vi "23384_Davis_Poku_Amankwa_Amankwa.DavisPoku.MNE1201.7.1_348263_723397803.vi"() -> ()   [LabVIEW 2018]
panel:
  out "C":bool
  out "B":bool
  out "E":bool
  out "D":bool
  out "G":bool
  out "F":bool
  out "A":bool
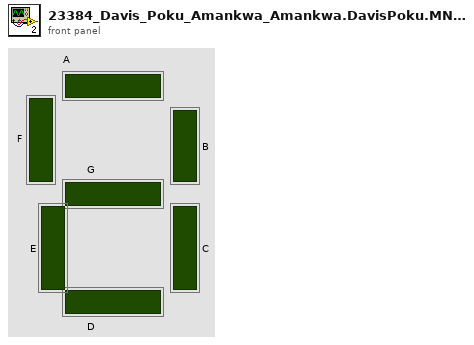
[diagram p1: front panel]
types:
  T1 = enum16{"0", "1", "2", "3", "4", "5", "6", "7", "8", "9", "OFF"}
  T2 = enum16{"0", "1", "2", "3", "4", "5", "6", "7", "8", "9"}
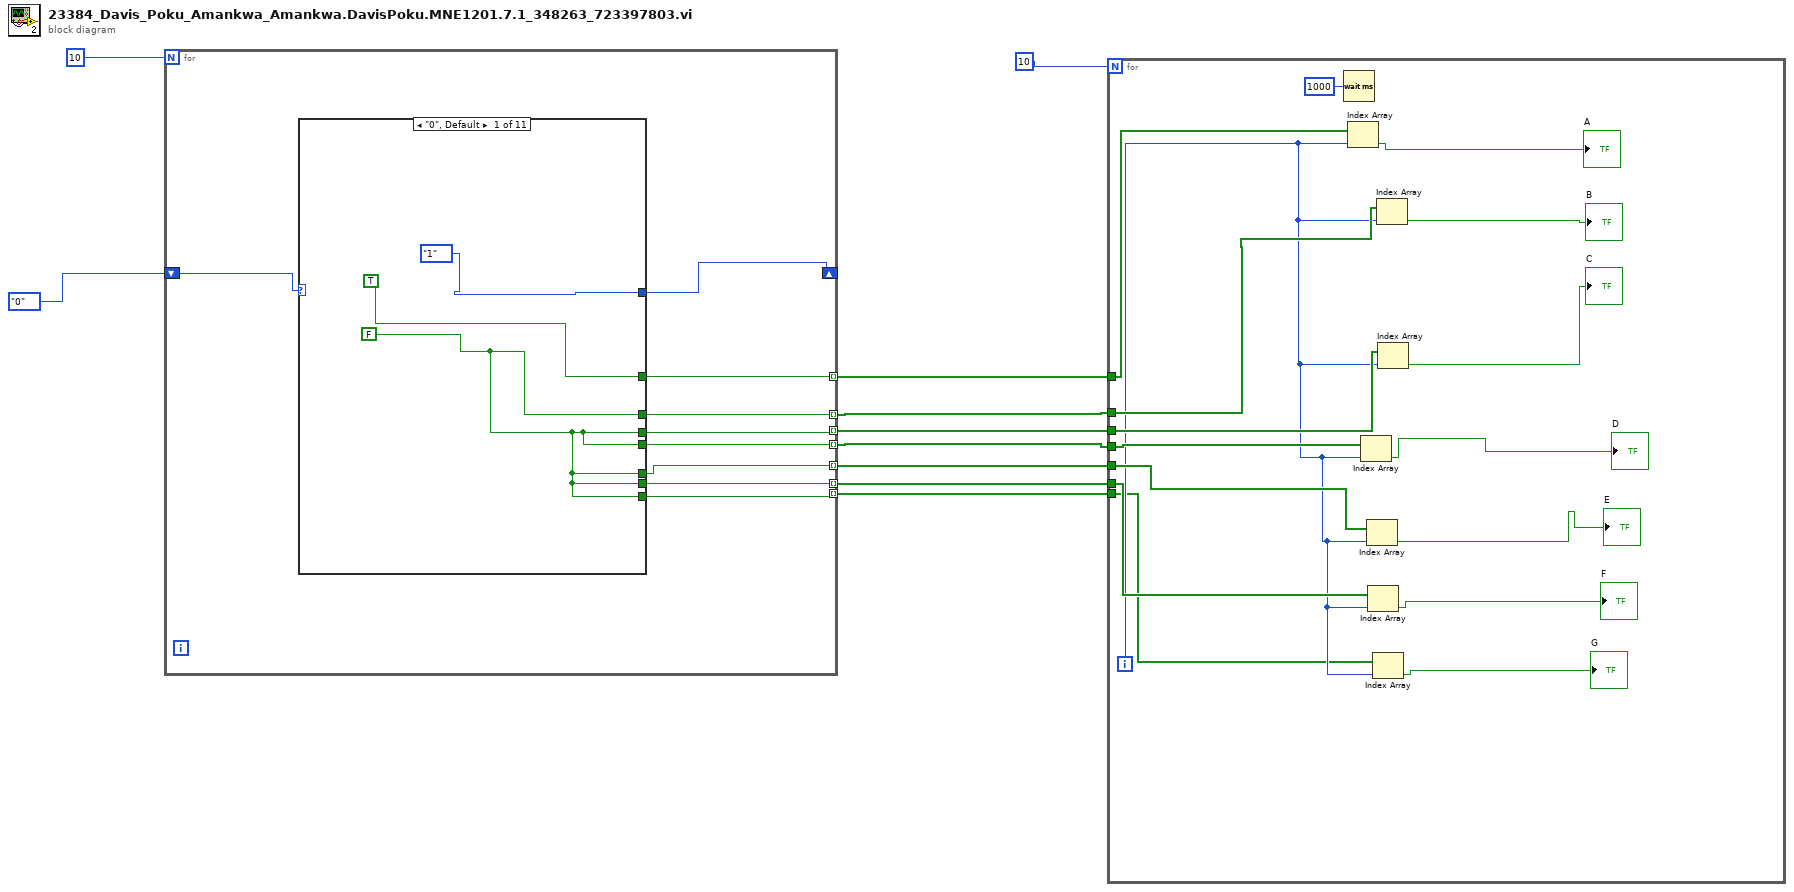
[diagram p0: block diagram]
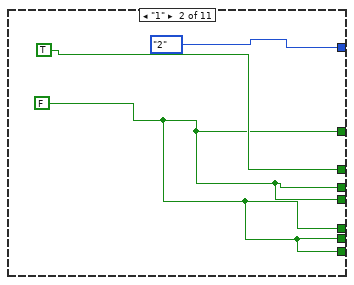
[diagram p2: hidden frame]
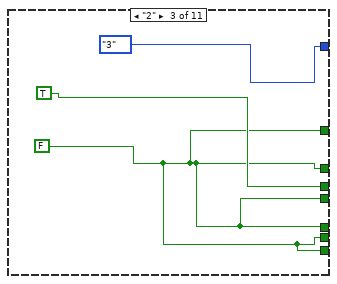
[diagram p3: hidden frame]
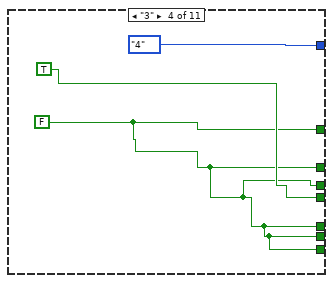
[diagram p4: hidden frame]
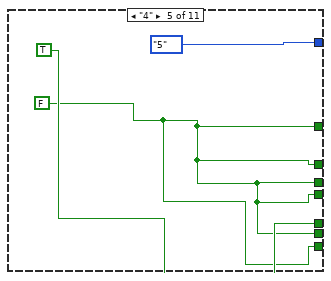
[diagram p5: hidden frame]
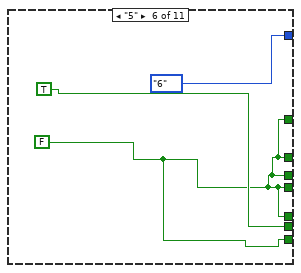
[diagram p6: hidden frame]
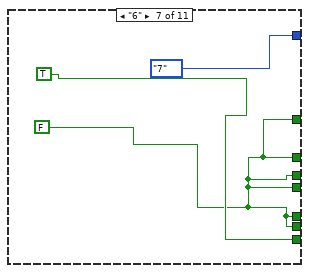
[diagram p7: hidden frame]
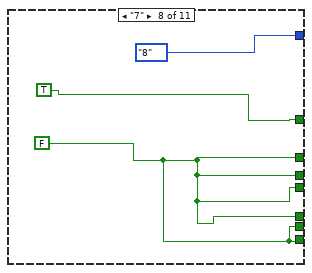
[diagram p8: hidden frame]
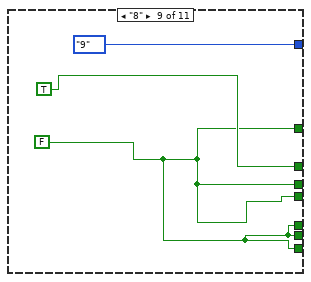
[diagram p9: hidden frame]
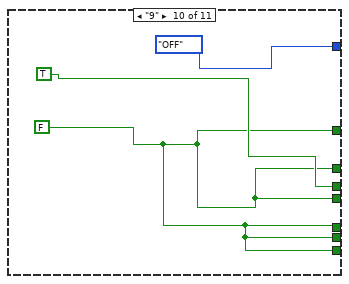
[diagram p10: hidden frame]
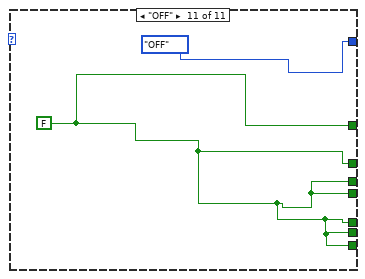
[diagram p11: hidden frame]
diagram:
  n1 = for {
    N: 10 -> [_]
    shift-right: [w19] -> _
    shift-left: T1."0" -> [w18]
    tunnel: [w17] -> w8 mode=indexing
    tunnel: [w16] -> w6 mode=indexing
    tunnel: [w15] -> w5 mode=indexing
    tunnel: [w14] -> w4 mode=indexing
    tunnel: [w13] -> w3 mode=indexing
    tunnel: [w12] -> w2 mode=indexing
    tunnel: [w11] -> w1 mode=indexing
    n2 = case shown="\"0\", Default" w18 {
      tunnel: [TRUE w23 w26 w29 w32 w35 w38 TRUE w45 w48 w51] -> w17
      tunnel: [w21 TRUE w26 w29 w32 w35 w38 w41 TRUE w48 w51] -> w16
      tunnel: [w21 w23 TRUE w29 w32 w35 w38 w41 w45 TRUE w51] -> w15
      tunnel: [w21 w23 w26 TRUE w32 w35 w38 w41 w45 w48 w51] -> w14
      tunnel: [w21 w23 w26 w29 TRUE w35 w38 w41 w45 w48 w51] -> w13
      tunnel: [w21 w23 w26 w29 w32 TRUE w38 w41 w45 w48 w51] -> w12
      tunnel: [w21 w23 w26 w29 w32 w35 TRUE w41 w45 w48 w51] -> w11
      tunnel: [T1."1" T2."2" T2."3" T2."4" T2."5" T2."6" T2."7" T2."8" T2."9" T1."OFF" T1."OFF"] -> w19
      frame "0", Default {
        w21 = FALSE
      }
      frame "1" {
        w23 = FALSE
      }
      frame "2" {
        w26 = FALSE
      }
      frame "3" {
        w29 = FALSE
      }
      frame "4" {
        w32 = FALSE
      }
      frame "5" {
        w35 = FALSE
      }
      frame "6" {
        w38 = FALSE
      }
      frame "7" {
        w41 = FALSE
      }
      frame "8" {
        w45 = FALSE
      }
      frame "9" {
        w48 = FALSE
      }
      frame "OFF" {
        w51 = FALSE
      }
    }
  }
  n3 = for {
    N: 10 -> [_]
    tunnel: w8 -> [w67]
    tunnel: w6 -> [w63]
    tunnel: w5 -> [w62]
    tunnel: w4 -> [w61]
    tunnel: w3 -> [w60]
    tunnel: w2 -> [w59]
    tunnel: w1 -> [w53]
    i -> [w54]
    n4 = Wait (ms)(milliseconds to wait=u32 1000) -> ()  [unwired: 1 out]
    n5 = Index Array(array=w67, index=w54) -> (element=→"A":bool)
    n6 = Index Array(array=w61, index=w54) -> (element=→"D":bool)
    n7 = Index Array(array=w60, index=w54) -> (element=→"E":bool)
    n8 = Index Array(array=w59, index=w54) -> (element=→"F":bool)
    n9 = Index Array(array=w53, index=w54) -> (element=→"G":bool)
    n10 = Index Array(array=w63, index=w54) -> (element=→"B":bool)
    n11 = Index Array(array=w62, index=w54) -> (element=→"C":bool)
  }
